vi "clear.vi"(7 "dvr":refnum<data-value>, 8 "error in (no error)":errorcluster) -> (0 "error out":errorcluster)   [LabVIEW 2015, in "lv-graph-global.lvlib"]
doc: "Preload can be used to store a data set in total. This can be used to \"load\" data from an alternate source rather than generating a set of points at a time."
uses:
  _controls/data.ctl
  _controls/configuration.ctl
  _controls/store_method.ctl
  lv-graph-global.lvlib
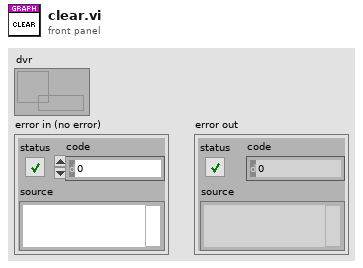
[diagram p1: front panel]
types:
  T1 = typedef "lv-graph-global.lvlib/data.ctl" = cluster{"configuration":T2, "index":i32, "x_axis":dbl[], "y_axis":dbl[][]}
  T2 = typedef "lv-graph-global.lvlib/configuration.ctl" = cluster{"store_method":T3, "rows":i32, "columns":i32}
  T3 = typedef "lv-graph-global.lvlib/store_method.ctl" = enum16{"<store_method>", "fixed", "grow"}
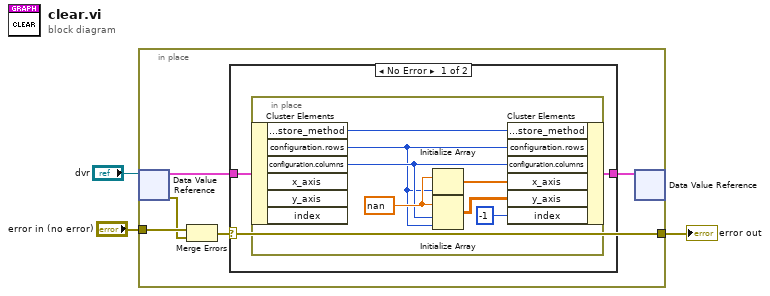
[diagram p0: block diagram]
diagram:
  n1 = in-place {
    in-place-border: "error in (no error)" -> [w8]
    in-place-border: [w4] -> w1
    n2 = in-place-dvr #1("dvr") -> (w6:T1, w7:errorcluster)
    n3 = Merge Errors(w8, w7) -> (w4:errorcluster)
    n4 = case shown="No Error" w4 {
      tunnel: w6 -> [w10 w18]
      tunnel: [w9 w18] -> w5
      frame No Error {
        n5 = in-place {
          w16 = nan
          n6 = in-place-cluster #2(w10) -> ("configuration.store_method"=w17:T3, "configuration.rows"=w14:i32, "configuration.columns"=w15:i32)  [unwired: 3 out]
          n7 = Initialize Array(w16, w14) -> (w13:dbl[])
          n8 = Initialize Array(w16, w15, w14) -> (w12:dbl[][])
          n9 = in-place-cluster #2("configuration.store_method"=w17, "configuration.rows"=w14, "configuration.columns"=w15, "x_axis"=w13, "y_axis"=w12, "index"=-1 ("Index")) -> (w9:T1)
        }
      }
      frame Error {
      }
    }
    n10 = in-place-dvr #1(w5) -> ()  [unwired: 2 out]
  }
  "error out" <- w1
